vi "HISW_2_PAQ1sec.vi"(8 "error in (no error)":errorcluster, 10 "PAQdatagram IN":T3 {"data" format="%.2f"; "status" format="%08x"}, 11 "AVPP in":refnum<class "AVPP.lvclass">) -> (0 "error out":errorcluster, 2 "Next_Level":T1, 3 "AVPP out":refnum<class "AVPP.lvclass">)   [LabVIEW 2020]
doc: "Process the Saving of 1 second samples towards the FAMM"
uses:
  AVPP.lvclass
  D:/Labview/Sgraph/Sgraph/source/FAMM/FAMM.lvclass
  HISW/controls/typedef_PAQdatagram.ctl
  FAMM/controls/typedef_AverageAction.ctl
  FAMM/controls/typedef_Level.ctl
  FAMM/controls/MemStoreDatagram.ctl
  FAMM/FAMM.lvclass
  HISW/HISW.lvclass
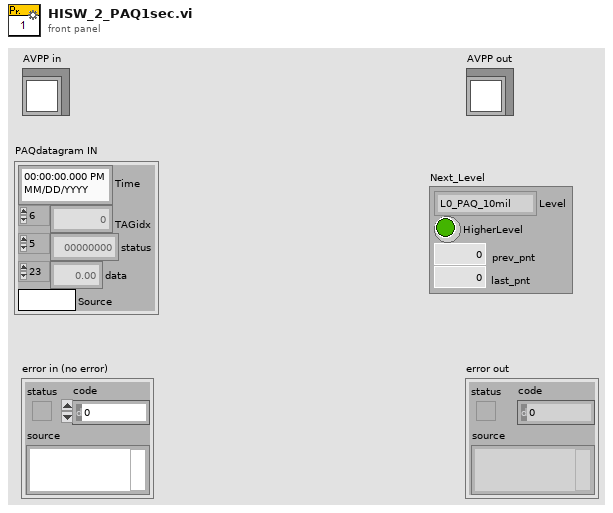
[diagram p1: front panel]
types:
  T1 = typedef "Sgraph_lib_V1.lvlib/FAMM.lvclass/typedef_AverageAction.ctl" = cluster{"Level":T2, "HigherLevel":bool, "prev_pnt":i32, "last_pnt":i32}
  T2 = typedef "Sgraph_lib_V1.lvlib/FAMM.lvclass/typedef_Level.ctl" = enum16{"L0_PAQ_10mil", "L0_PAQ_100mil", "L1_PAQ_100mil", "L2_PAQ_1sec", "L3_PAQ_10sec", "L4_PAQ_1min", "L5_PAQ_10min", "L6_PAQ_2hr", "L7_PAQ_1day", "L8_PAQ_1wk", "L1_PAQ_1sec", "L2_PAQ_10sec", "L3_PAQ_1min", "L4_PAQ_10min", "L5_PAQ_2hr", "L6_PAQ_1day", "L7_PAQ_1wk", "L0_PAQ_1sec", "L1_PAQ_10sec", "L2_PAQ_1min", "L3_PAQ_10min", "L4_PAQ_2hr", "L5_PAQ_1day", "L6_PAQ_1wk", "L0_PAQ_10sec", "L1_PAQ_1min", "L2_PAQ_10min", "L3_PAQ_2hr", "L4_PAQ_1day", "L5_PAQ_1wk"}
  T3 = typedef "typedef_PAQdatagram.ctl" = cluster{"Time":timestamp, "TAGidx":i32[], "status":u32[], "data":dbl[], "Source":string}
  T4 = typedef "Sgraph_lib_V1.lvlib/FAMM.lvclass/MemStoreDatagram.ctl" = cluster{"Time":dbl, "TagIndex":i32[], "data":dbl[], "max":dbl[], "min":dbl[], "status":u32[], "Source":string}
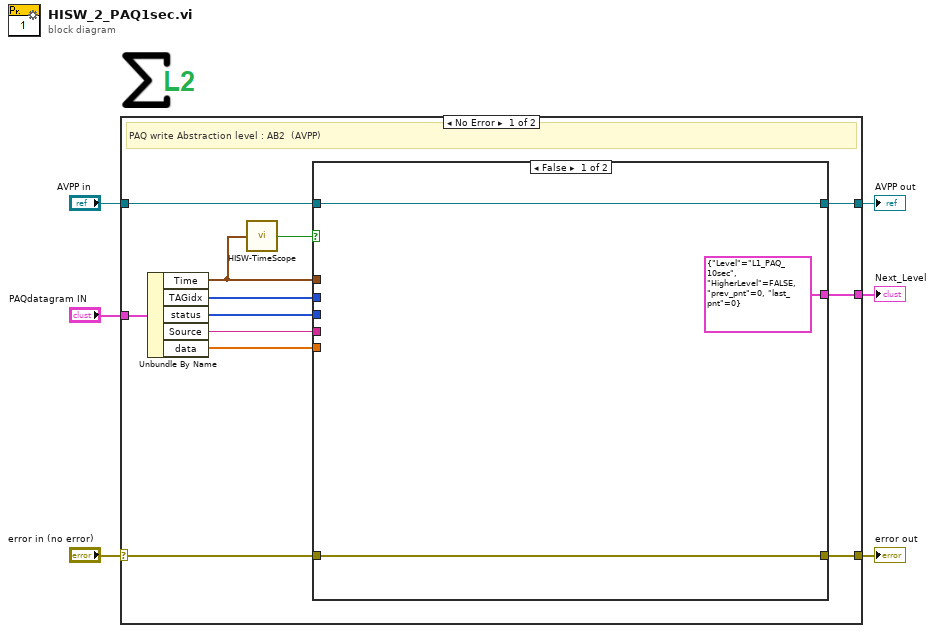
[diagram p0: block diagram]
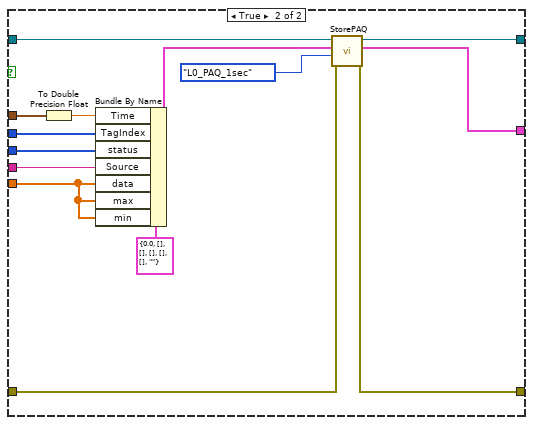
[diagram p2: hidden frame]
diagram:
  n1 = case shown="No Error" "error in (no error)" {
    selector: "error in (no error)" -> [w11 w37]
    tunnel: [w10 w37] -> w5
    tunnel: [w18 w36] -> w3
    tunnel: "AVPP in" -> [w15 w36]
    tunnel: "PAQdatagram IN" -> [w17 _]
    tunnel: [w9 _] -> w1
    frame No Error {
      # "PAQ write Abstraction level : AB2  (AVPP)"
      n2 = Unbundle By Name(w17) -> ("Time"=w8:timestamp, "TAGidx"=w16:i32[], "status"=w14:u32[], "Source"=w13:string, "data"=w12:dbl[])
      n3 = call "HISW-TimeScope.vi"("Time"=w8) -> ("Valid?"=w7:bool)  [unwired: 8 in]
      n4 = case shown="False" w7 {
        tunnel: [w21 w35] -> w18
        tunnel: w16 -> [_ w32]
        tunnel: w15 -> [w21 w31]
        tunnel: w14 -> [_ w30]
        tunnel: w13 -> [_ w29]
        tunnel: w12 -> [_ w27]
        tunnel: w11 -> [w20 w26]
        tunnel: [w20 w25] -> w10
        tunnel: [T1 {"Level"=enum."L1_PAQ_10sec", "HigherLevel"=FALSE, "prev_pnt"=0, "last_pnt"=0} ("Next_Level") w23] -> w9
        tunnel: w8 -> [_ w22]
        frame False {
        }
        frame True {
          n5 = To Double Precision Float(number=w22) -> (double precision float=w33:dbl)
          n6 = Bundle By Name(cluster=T4 {"Time"=0.0, "TagIndex"=[], "data"=[], "max"=[], "min"=[], "status"=[], "Source"=""} ("StoreDatagram"), "Time"=w33, "TagIndex"=w32, "status"=w30, "Source"=w29, "data"=w27, "max"=w27, "min"=w27) -> (w28:T4)
          n7 = call "StorePAQ.vi"("error in (no error)"=w26, "Level"=typedef_Level."L0_PAQ_1sec" ("Enum"), "StoreDatagram"=w28, "FAMM in"=w31) -> ("error out"=w25:errorcluster, "Next_Level"=w23:T1, "FAMM out"=w35:refnum<class "AVPP.lvclass">)  [unwired: 5 in]
        }
      }
    }
    frame Error {
    }
  }
  "error out" <- w5
  "AVPP out" <- w3
  "Next_Level" <- w1
